vi "DSF.Engine.Execution.Builder.New.vi"(8 "error in (no error)":errorcluster, 10 "Framework Cache":refnum<class "DSF.Engine.Memory.Cache.Framework.lvclass">, 11 "Plugin Buffer Pools":refnum<class "DSF.Engine.Memory.BufferPool.lvclass">[](array[class])) -> (0 "error out":errorcluster, 3 "Builder":refnum<class "DSF.Engine.Execution.Builder.lvclass">)   [LabVIEW 2016, in "DSF.Engine.lvlib" / "DSF.Engine.Execution.Builder.lvclass"]
uses:
  Builder/DSF.Engine.Execution.Builder.lvclass
  BufferPool/DSF.Engine.Memory.BufferPool.lvclass
  Cache/DSF.Engine.Memory.Cache.Framework.lvclass
  DSF.Engine.Execution.Builder.FIFOs.ctl
  DSF.Engine.Execution.Builder.Command FIFO.ctl
  DSF.Engine.Execution.Builder.Command Payload.ctl
  DSF.Engine.Execution.Builder.Commands.ctl
  DSF.Engine.Execution.Builder.Response FIFO.ctl
  DSF.Engine.Execution.Builder.Response Payload.ctl
  Builder/DSF.Engine.Execution.Builder.lvclass/DSF.Engine.Execution.Builder.ctl
  DSF.Engine.Execution.Builder.Status Pointers.ctl
  Memory.Pointer/DSF.Memory.Pointer.U32.lvclass
  C:/Git/Sourcetree/DSF/Source/Submodules/Memory Manager/Source/Classes/Pointer.Internal/Memory.Pointer.Internal.lvclass
  Submodules/Memory Manager/Source/Classes/Pointer.Internal/Methods/Memory.Pointer.Internal.Allocate.vi
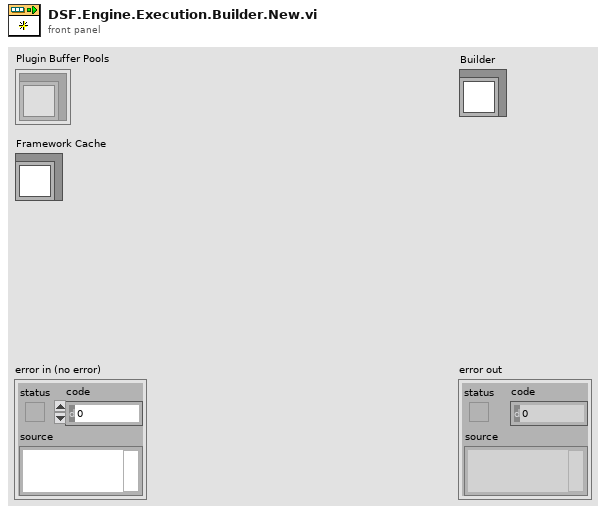
[diagram p1: front panel]
types:
  T1 = typedef "DSF.Engine.lvlib/DSF.Engine.Execution.Builder.lvclass/DSF.Engine.Execution.Builder.Status Pointers.ctl" = cluster{"Build Duration":refnum<class "DSF.Memory.Pointer.U32.lvclass">}
  T2 = typedef "DSF.Engine.lvlib/DSF.Engine.Execution.Builder.lvclass/DSF.Engine.Execution.Builder.Response Payload.ctl" = cluster{"command":T3}
  T3 = typedef "DSF.Engine.lvlib/DSF.Engine.Execution.Builder.lvclass/DSF.Engine.Execution.Builder.Commands.ctl" = enum8{"Initialize", "Build", "Parse", "Shutdown"}
  T4 = cluster{"read mode":enum16{"polling", "blocking"}, "write mode":enum16{"polling", "blocking"}}
  T5 = typedef "DSF.Engine.lvlib/DSF.Engine.Execution.Builder.lvclass/DSF.Engine.Execution.Builder.Command Payload.ctl" = cluster{"Command":T3, "Plugin ID":i32, "Transfer ID":i32}
  T6 = typedef "DSF.Engine.lvlib/DSF.Engine.Execution.Builder.lvclass/DSF.Engine.Execution.Builder.FIFOs.ctl" = cluster{"Command FIFO":T7, "Response FIFO":T8}
  T7 = typedef "DSF.Engine.lvlib/DSF.Engine.Execution.Builder.lvclass/DSF.Engine.Execution.Builder.Command FIFO.ctl" = refnum<k33>
  T8 = typedef "DSF.Engine.lvlib/DSF.Engine.Execution.Builder.lvclass/DSF.Engine.Execution.Builder.Response FIFO.ctl" = refnum<k33>
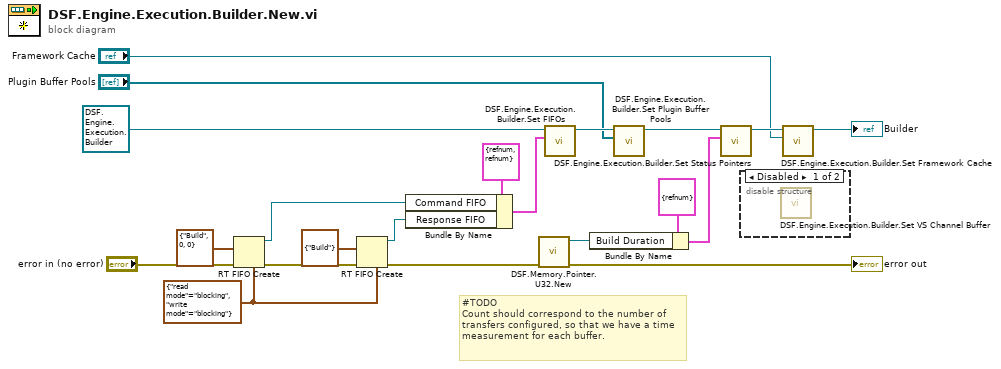
[diagram p0: block diagram]
diagram:
  w13 = T4 {"read mode"=enum."blocking", "write mode"=enum."blocking"} ("r/w modes (polling,polling)")
  # "#TODO\nCount should correspond to the number of transfers configured, so that we have a time measurement for each buffer."
  n1 = RT FIFO Create(1:T5 {"Command"=enum."Build", "Plugin ID"=0, "Transfer ID"=0} ("Command Payload"), 3:"error in (no error)", 7:w13) -> (8:w11:refnum<k33>, 11:w14:errorcluster)  [unwired: 5 in, 1 out]
  n2 = RT FIFO Create(1:T2 {"command"=enum."Build"} ("Response Payload"), 3:w14, 7:w13) -> (8:w10:refnum<k33>, 11:w8:errorcluster)  [unwired: 5 in, 1 out]
  n3 = Bundle By Name(cluster=T6 {"Command FIFO"=refnum, "Response FIFO"=refnum} ("FIFOs"), "Command FIFO"=w11, "Response FIFO"=w10) -> (w17:T6)
  n4 = call "DSF.Memory.Pointer.U32.New.vi"("error in (no error)"=w8) -> ("error out"=→"error out":errorcluster, "pointer"=w6:refnum<class "DSF.Memory.Pointer.U32.lvclass">)  [unwired: 9 in]
  n5 = call "DSF.Engine.Execution.Builder.Set FIFOs.vi"("FIFOs"=w17, "Builder in"=refnum<class "DSF.Engine.Execution.Builder.lvclass"> refnum ("Builder")) -> ("Builder out"=w20:refnum<class "DSF.Engine.Execution.Builder.lvclass">)  [unwired: 8 in, 1 out]
  n6 = Bundle By Name(cluster=T1 {"Build Duration"=refnum} ("Status Pointers"), "Build Duration"=w6) -> (w5:T1)
  n7 = call "DSF.Engine.Execution.Builder.Set Plugin Buffer Pools.vi"("Plugin Buffer Pools"="Plugin Buffer Pools", "Builder in"=w20) -> ("Builder out"=w19:refnum<class "DSF.Engine.Execution.Builder.lvclass">)  [unwired: 8 in, 1 out]
  n8 = call "DSF.Engine.Execution.Builder.Set Status Pointers.vi"("Status Pointers"=w5, "Builder in"=w19) -> ("Builder out"=w3:refnum<class "DSF.Engine.Execution.Builder.lvclass">)  [unwired: 8 in, 1 out]
  n9 = disable-structure shown="Disabled" {
    frame Disabled {
      n10 = call "DSF.Engine.Execution.Builder.Set VS Channel Buffer.vi"() -> ()  [unwired: 10 in, 2 out]
    }
    frame Enabled {
    }
  }
  n11 = call "DSF.Engine.Execution.Builder.Set Framework Cache.vi"("Framework Cache"="Framework Cache", "Builder in"=w3) -> ("Builder out"=→"Builder":refnum<class "DSF.Engine.Execution.Builder.lvclass">)  [unwired: 8 in, 1 out]
